vi "CRC.vi"(9 "Polynomial":u8=7, 10 "ResetValue":u8=255, 11 "Data":u8[](array[numeric])) -> (3 "CRC8":u8=49)   [LabVIEW 2009]
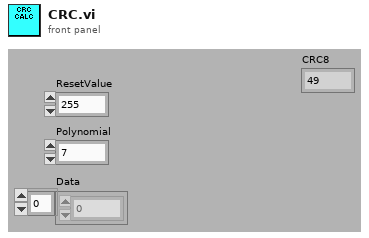
[diagram p1: front panel]
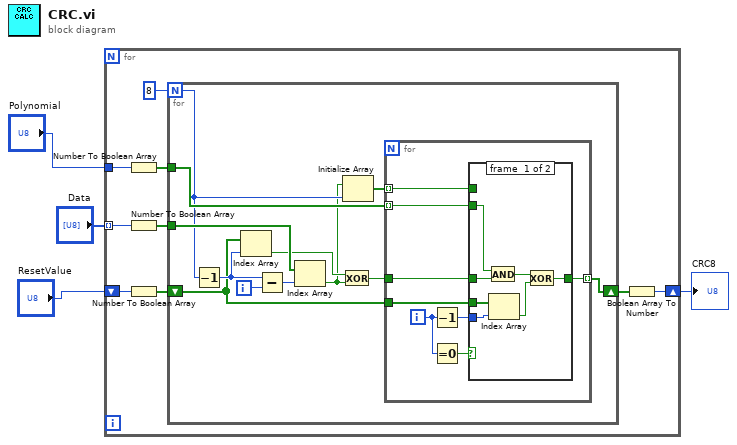
[diagram p0: block diagram]
diagram:
  n1 = for {
    tunnel: "Data" -> [w13] mode=indexing
    shift-right: [w10] -> w3
    shift-left: "ResetValue" -> [w5]
    tunnel: "Polynomial" -> [w7]
    n2 = Number To Boolean Array(number=w7) -> (Boolean array=w6:bool[])
    n3 = Number To Boolean Array(number=w13) -> (Boolean array=w11:bool[])
    n4 = Number To Boolean Array(number=w5) -> (Boolean array=w9:bool[])
    n5 = for {
      N: 8 -> [w18]
      tunnel: w11 -> [w24]
      shift-right: [w15] -> w8
      shift-left: w9 -> [w14]
      tunnel: w6 -> [w19]
      i -> [w25]
      n6 = Decrement(x=w18) -> (x-1=w22:i32)
      n7 = Index Array(array=w14, index=w22) -> (element=w21:bool)
      n8 = Subtract(x=w22, y=w25) -> (x-y=w23:i32)
      n9 = Index Array(array=w24, index=w23) -> (element=w17:bool)
      n10 = Exclusive Or(1:w17, 2:w21) -> (0:w20:bool)
      n11 = Initialize Array(w17, w18) -> (w16:bool[])
      n12 = for {
        tunnel: w20 -> [w30]
        tunnel: w19 -> [w26] mode=indexing
        tunnel: w16 -> [w32] mode=indexing
        tunnel: [w31] -> w15 mode=indexing
        tunnel: w14 -> [w29]
        i -> [w28]
        n13 = Decrement(x=w28) -> (x-1=w27:i32)
        n14 = Equal To 0?(x=w28) -> (x = 0?=w33:bool)
        n15 = case shown="False" w33 {
          tunnel: w32 -> [_ _]
          tunnel: [w34 w41] -> w31
          tunnel: w30 -> [w38 w41]
          tunnel: w29 -> [w40 _]
          tunnel: w27 -> [w39 _]
          tunnel: w26 -> [w37 _]
          frame #0 {
            n16 = And(x=w37, y=w38) -> (x .and. y?=w36:bool)
            n17 = Index Array(array=w40, index=w39) -> (element=w35:bool)
            n18 = Exclusive Or(1:w35, 2:w36) -> (0:w34:bool)
          }
          frame #1 {
          }
        }
      }
    }
    n19 = Boolean Array To Number(Boolean array=w8) -> (number=w10:u32)
  }
  "CRC8" <- w3
